vi "FdxProcessMonQueueCvi.vi"(8 "error in":errorcluster, 11 "MonQueue":cluster{"ReadQualifier":u32, "Entries":u32} {"ReadQualifier" items=["FDX_MON_READ_FULL", "FDX_MON_READ_HEADER", "FDX_MON_READ_DATA"]}) -> (0 "error out":errorcluster, 9 "MonQueueData":u8[](array[numeric]))   [LabVIEW 2020, in "AIM664LV.lvlib"]
doc: "This function processes data, read via AiFdxCmdMonQueueRead in order to the Frame Header Information. The processing mainly affects platform dependent variable interpretation / structure access (Little/Big Endian) of the Frame Header Information. Frame Data remains unchanged. This function is typcially used in conjunction with AiFdxCmdMonQueueRead function.\nNote: Data, read via AiFdxCmdMonQueueRead (without processing via this function) can be directly used for Replay via the AiFdxCmdTxQueueWrite function, if the corresponding Transmit Port has been configured for Replay. This avoids any data processing when using previously captured traffic for Replay."
uses:
  AIM664LV.lvlib
  AFDX_LibraryAdmin/FdxGlobalDllPath.vi
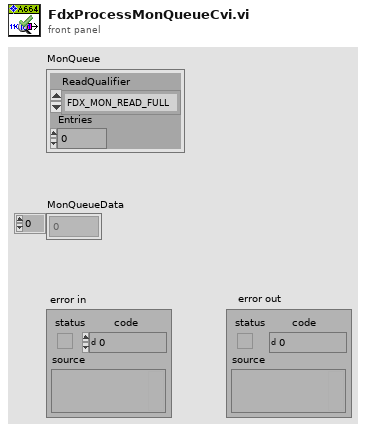
[diagram p1: front panel]
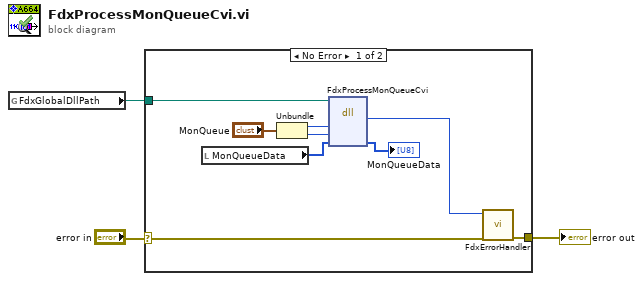
[diagram p0: block diagram]
diagram:
  n1 = global read "FdxGlobalDllPath.vi" "FdxGlobalDllPath"() -> (w1:path)
  n2 = case shown="No Error" "error in" {
    selector: "error in" -> [w11 w13]
    tunnel: [w12 w13] -> w3
    tunnel: w1 -> [w4 _]
    frame No Error {
      n3 = local read "MonQueueData"() -> (w5:u8[])
      n4 = Unbundle("MonQueue") -> ("ReadQualifier"=w7:u32, "Entries"=w6:u32)
      n5 = dll-call lib="aim_fdx.19.dll" fn="FdxProcessMonQueueCvi"(path in=w4, "ReadQualifier"=w7, "Entries"=w6, "MonQueueData"=w5) -> ("status"=w10:i32, "MonQueueData"=→"MonQueueData":u8[])  [unwired: 4 in, 2 out]
      n6 = call "FdxErrorHandler.vi"("error in"=w11, "AIM Error"=w10) -> ("error out"=w12:errorcluster)  [unwired: 9 in]
    }
    frame Error {
    }
  }
  "error out" <- w3
